vi "host_cmd_ini.vi"(8 "error in (no error)":errorcluster) -> (0 "error out":errorcluster)   [LabVIEW 2021]
doc: "This VI initialize variables for command. The counter for move will reset to 0."
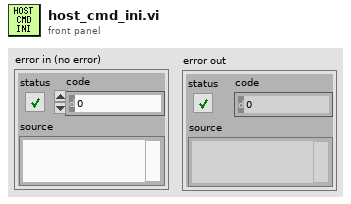
[diagram p1: front panel]
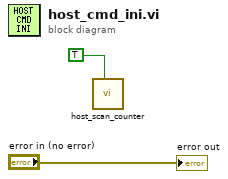
[diagram p0: block diagram]
diagram:
  n1 = call "host_scan_counter.vi"("reset?"=TRUE) -> ()  [unwired: 10 in, 1 out]
  "error out" <- "error in (no error)"
